vi "IVsweep.vi"(4 "Dwell time":u32, 5 "Npoints":i32=20, 6 "Vstop":dbl=1.0, 7 "Vstart":dbl, 8 "Device":u8=1, 9 "Serial port":refnum<visa-resource-name>) -> (0 "Current":sgl[](array[numeric]), 1 "Voltage":dbl[](array[numeric]), 2 "Device out":u8=1, 3 "Serial port out":refnum<visa-resource-name>)   [LabVIEW 2021]
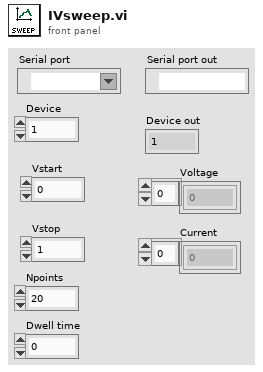
[diagram p1: front panel]
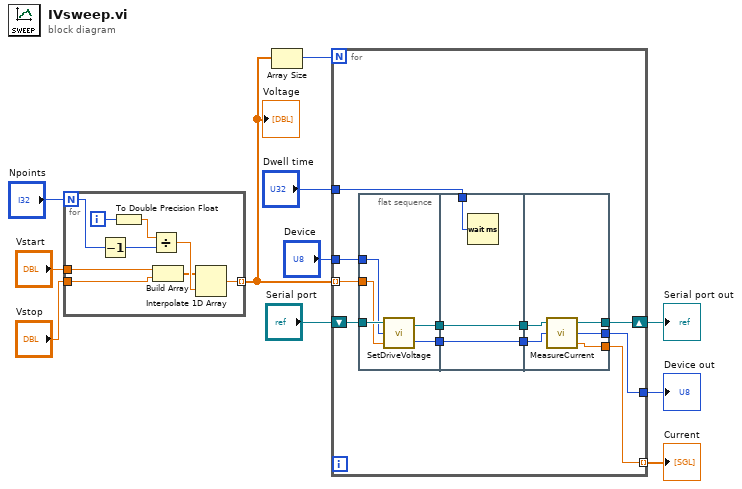
[diagram p0: block diagram]
diagram:
  n1 = for {
    N: "Npoints" -> [w16]
    tunnel: [w17] -> w7 mode=indexing
    tunnel: "Vstart" -> [w14]
    tunnel: "Vstop" -> [w13]
    i -> [w20]
    n2 = Decrement(x=w16) -> (x-1=w15:i32)
    n3 = To Double Precision Float(number=w20) -> (double precision float=w19:dbl)
    n4 = Divide(x=w19, y=w15) -> (x/y=w18:dbl)
    n5 = Build Array(w14, w13) -> (w12:dbl[])
    n6 = Interpolate 1D Array(1:w18, 2:w12) -> (0:w17:dbl)
  }
  "Voltage" <- w7
  n7 = Array Size(array=w7) -> (size(s)=w8:i32)
  n8 = for {
    N: w8 -> [_]
    tunnel: w7 -> [w27] mode=indexing
    tunnel: "Dwell time" -> [w31]
    tunnel: "Device" -> [w24]
    shift-right: [w26] -> w4
    shift-left: "Serial port" -> [w28]
    tunnel: [w25] -> w2 mode=indexing
    tunnel: [w21] -> w1
    n9 = flat-sequence {
      tunnel: [w36] -> w29
      tunnel: w28 -> [w35]
      tunnel: w27 -> [w34]
      tunnel: w24 -> [w33]
      tunnel: [w32] -> w22
      tunnel: w31 -> [w39]
      tunnel: [w38] -> w30
      tunnel: w29 -> [w38]
      tunnel: [w37] -> w23
      tunnel: w22 -> [w37]
      tunnel: w30 -> [w44]
      tunnel: [w43] -> w26
      tunnel: [w42] -> w25
      tunnel: w23 -> [w41]
      tunnel: [w40] -> w21
      frame #0 {
        n10 = call "SetDriveVoltage.vi"("Voltage"=w34, "Device"=w33, "Serial port"=w35) -> ("Device out"=w32:u8, "Serial port out"=w36:refnum<visa-resource-name>)
      }
      frame #1 {
        n11 = Wait (ms)(milliseconds to wait=w39) -> ()  [unwired: 1 out]
      }
      frame #2 {
        n12 = call "MeasureCurrent.vi"("Device"=w41, "Serial port"=w44) -> ("Current"=w42:sgl, "Device out"=w40:u8, "Serial port out"=w43:refnum<visa-resource-name>)  [unwired: 1 in]
      }
    }
  }
  "Current" <- w2
  "Serial port out" <- w4
  "Device out" <- w1
